vi "Destroy.vi"(8 "Error In":errorcluster, 11 "reference in":refnum<class "VdDigitalControl_DAQmx.lvclass">) -> (0 "Error Out":errorcluster, 3 "reference out":refnum<class "VdDigitalControl_DAQmx.lvclass">)   [LabVIEW 2020, in "VdDigitalControl_DAQmx.lvclass"]
uses:
  VdDigitalControl_DAQmx.lvclass
  VdDigitalControl_DAQmx.lvclass/VdDigitalControl_DAQmx.ctl
  VdDigitalControl_class/VdDigitalControl.lvclass
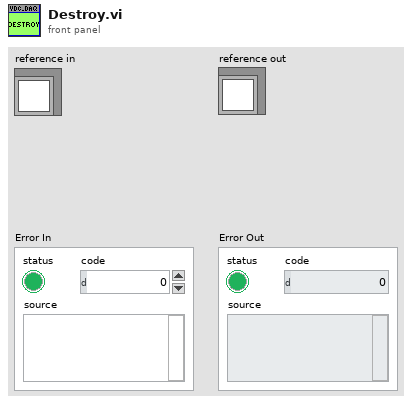
[diagram p1: front panel]
types:
  T1 = typedef "VdDigitalControl_DAQmx.lvclass/ObjectAttributes.ctl" = cluster{"task":refnum<k21>}
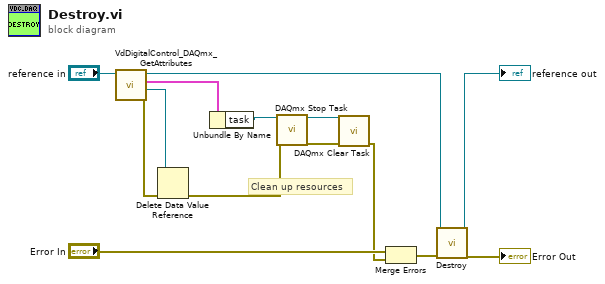
[diagram p0: block diagram]
diagram:
  # "Clean up resources"
  n1 = call "VdDigitalControl_DAQmx_GetAttributes.vi"("reference in"="reference in") -> ("error out"=w12:errorcluster, "DataRef"=w9:refnum<data-value>, "Data"=w11:T1, "reference out"=w10:refnum<class "VdDigitalControl_DAQmx.lvclass">)  [unwired: 7 in]
  n2 = Delete Data Value Reference(data value reference=w9, error in=w12) -> (error out=w3:errorcluster)  [unwired: 1 out]
  n3 = Unbundle By Name(w11) -> ("task"=w4:refnum<k21>)
  n4 = call <vilib>:"DAQmx Stop Task.vi"("task/channels in"=w4, "error in"=w3) -> ("task out"=w1:refnum<k21>, "error out"=w5:errorcluster)  [unwired: 12 in]
  n5 = call <vilib>:"DAQmx Clear Task.vi"("task in"=w1, "error in"=w5) -> ("error out"=w2:errorcluster)  [unwired: 13 in]
  n6 = Merge Errors("Error In", w2) -> (w14:errorcluster)
  n7 = call-parent "Destroy.vi"("Error In"=w14, "reference in"=w10) -> ("Error Out"=→"Error Out":errorcluster, "reference out"=→"reference out":refnum<class "VdDigitalControl_DAQmx.lvclass">)  [unwired: 8 in]
